vi "Security.FG.vi"(7 "Action":T1, 8 "error in (no error)":errorcluster, 10 "Security":T2={"Type"=enum."None", "Source DLL Path"=path "", "Target DLL Path"=path "", "Security Level"=1}, 11 "Device Item Ref in":T4 format="%.0x") -> (0 "error out":errorcluster, 2 "Security":T2={"Type"=enum."None", "Source DLL Path"=path "", "Target DLL Path"=path "", "Security Level"=1}, 3 "Device Item Ref out":T4=18446744073709551615 format="%.0x")   [LabVIEW 2019, in "Diagnostics Addon System Explorer.lvlib"]
uses:
  Diagnostics Addon System Explorer.lvlib
  <vilib>/NI VeriStand/Custom Device API/Custom Device Item Ref.ctl
  Shared/Types/Security.ctl
  Shared/Types/Security.Type.ctl
  Types/FG.Action.ctl
  Shared/SubVIs/Constants.vi
  <vilib>/NI VeriStand/Custom Device API/Get Item Property (U32).vi
  <vilib>/Utility/MD5Checksum.llb/MD5Checksum File.vi
  <vilib>/NI/NI VeriStand Advanced SysDef API/_SubVIs/SysDef.Property.Set.DependentFile.vi
  <vilib>/NI/NI VeriStand Advanced SysDef API/SysDef API/SysDef.Property.Remove.vi
  <vilib>/NI/NI VeriStand Advanced SysDef API/_SubVIs/SysDef.Property.Set.U32.vi
  Shared/Diagnostics Addon Shared.lvlib
  <vilib>/NI VeriStand/Custom Device API/Custom Device API.lvlib
  <vilib>/NI/NI VeriStand Advanced SysDef API/SysDef API/Advanced System Definition.lvlib
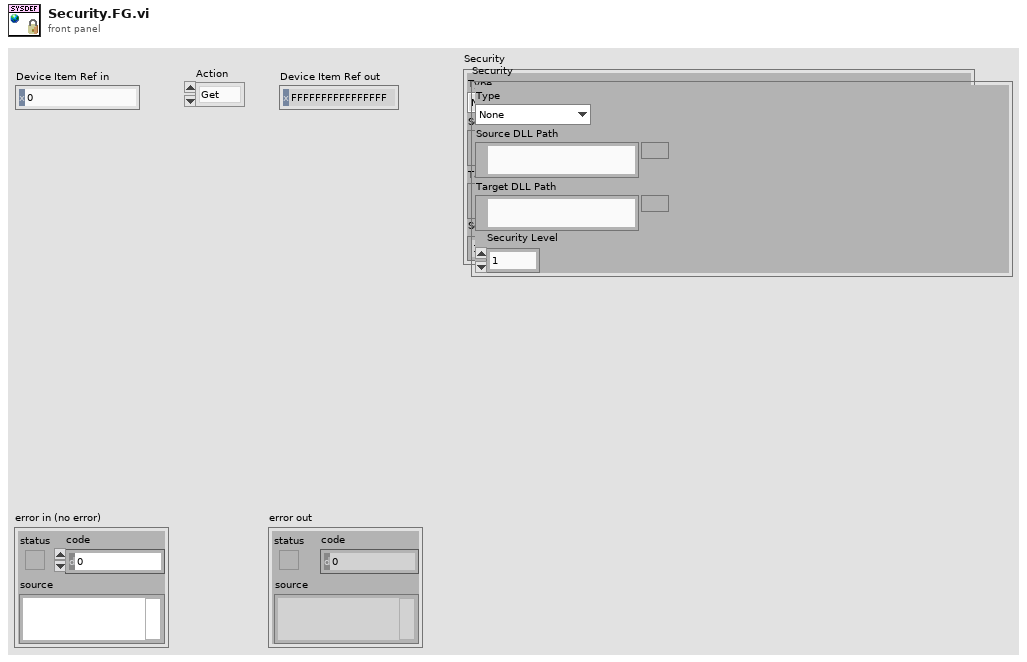
[diagram p1: front panel]
types:
  T1 = typedef "Diagnostics Addon System Explorer.lvlib/FG.Action.ctl" = enum16{"Get", "Set"}
  T2 = typedef "Diagnostics Addon Shared.lvlib/Security.ctl" = cluster{"Type":T3, "Source DLL Path":path, "Target DLL Path":path, "Security Level":u8}
  T3 = typedef "Diagnostics Addon Shared.lvlib/Security.Type.ctl" = enum16{"None", "DLL", "MasterKey"}
  T4 = typedef "Custom Device API.lvlib/Custom Device Item Ref.ctl" = u64
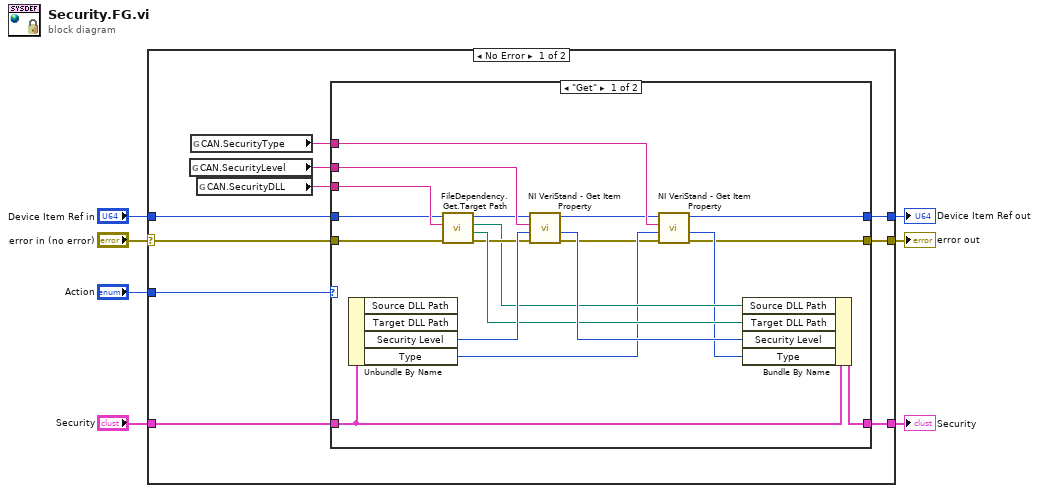
[diagram p0: block diagram]
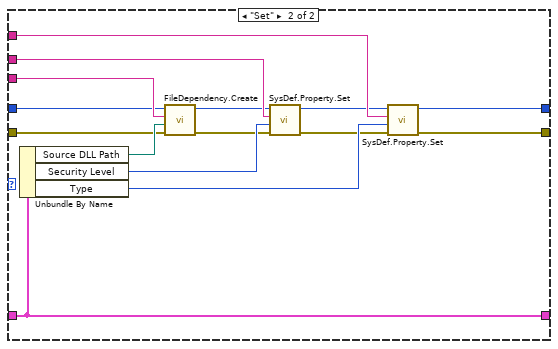
[diagram p2: hidden frame]
diagram:
  n1 = case shown="No Error" "error in (no error)" {
    selector: "error in (no error)" -> [w17 w52]
    tunnel: "Device Item Ref in" -> [w16 w53]
    tunnel: [w8 w53] -> w4
    tunnel: [w9 w52] -> w5
    tunnel: [w15 _] -> w3
    tunnel: "Security" -> [w14 _]
    tunnel: "Action" -> [w13 _]
    frame No Error {
      n2 = global read "Constants.vi" "CAN.SecurityLevel"() -> (w11:string)
      n3 = global read "Constants.vi" "CAN.SecurityType"() -> (w10:string)
      n4 = global read "Constants.vi" "CAN.SecurityDLL"() -> (w12:string)
      n5 = case shown="\"Get\"" w13 {
        tunnel: w17 -> [w23 w41]
        tunnel: w16 -> [w22 w42]
        tunnel: [w35 w51] -> w15
        tunnel: w14 -> [w36 w51]
        tunnel: w12 -> [w31 w46]
        tunnel: w11 -> [w32 w49]
        tunnel: w10 -> [w26 w44]
        tunnel: [w19 w38] -> w9
        tunnel: [w18 w37] -> w8
        frame "Get" {
          n6 = Unbundle By Name(w36) -> ("Security Level"=w34:u8, "Type"=w24:T3)  [unwired: 2 out]
          n7 = call "FileDependency.Get.Target Path.vi"("error in (no error)"=w23, "Bitfile 986x"=w31, "Item Ref in"=w22) -> ("error out"=w29:errorcluster, "Target Path"=w30:path, "Source Path"=w27:path, "Item Ref out"=w28:T4)  [unwired: 5 in]
          n8 = call-poly <vilib>:"NI VeriStand - Get Item Property.vi"("error in (no error)"=w29, "Default Value"=w34, "Property Name"=w32, "Item Ref in"=w28) -> ("error out"=w21:errorcluster, "Value"=w33:u32, "Item Ref out"=w20:T4)  [unwired: 4 in, 1 out]
          n9 = call-poly <vilib>:"NI VeriStand - Get Item Property.vi"("error in (no error)"=w21, "Default Value"=w24, "Property Name"=w26, "Item Ref in"=w20) -> ("error out"=w19:errorcluster, "Value"=w25:u32, "Item Ref out"=w18:T4)  [unwired: 4 in, 1 out]
          n10 = Bundle By Name(cluster=w36, "Source DLL Path"=w27, "Target DLL Path"=w30, "Security Level"=w33, "Type"=w25) -> (w35:T2)
        }
        frame "Set" {
          n11 = Unbundle By Name(w51) -> ("Source DLL Path"=w45:path, "Security Level"=w50:u8, "Type"=w43:T3)
          n12 = call "FileDependency.Create.vi"("error in (no error)"=w41, "DLL Path"=w45, "DLL Property Name"=w46, "Item Ref in"=w42) -> ("error out"=w48:errorcluster, "Item Ref out"=w47:T4)  [unwired: 6 in]
          n13 = call-poly <vilib>:"SysDef.Property.Set.vi"("error in (no error)"=w48, "Value"=w50, "Property Name"=w49, "nodeID"=w47) -> ("error out"=w40:errorcluster, "nodeID out"=w39:u64)  [unwired: 6 in]
          n14 = call-poly <vilib>:"SysDef.Property.Set.vi"("error in (no error)"=w40, "Value"=w43, "Property Name"=w44, "nodeID"=w39) -> ("error out"=w38:errorcluster, "nodeID out"=w37:u64)  [unwired: 6 in]
        }
      }
    }
    frame Error {
    }
  }
  "error out" <- w5
  "Device Item Ref out" <- w4
  "Security" <- w3
